vi "AssetMgrChangeHardwareForDeviceRequest_Parse.vi"(8 "error in (no error)":errorcluster, 11 "Message":T17) -> (0 "error out":errorcluster, 1 "Body":T1, 2 "Header":T16, 3 "AssetMgrChangeHardwareForDeviceRequest":T15)   [LabVIEW 2017]
uses:
  <vilib>/addons/InsightCM/MessageBus/Base/controls/Message.ctl
  <vilib>/addons/InsightCM/MessageBus/Base/controls/MessageHeader.ctl
  <vilib>/addons/InsightCM/MessageBus/Base/controls/KeyValuePair.ctl
  <vilib>/addons/InsightCM/MessageBus/MessageLibrary/AssetManager/controls/AssetMgrChangeHardwareForDeviceRequest.ctl
  <vilib>/addons/InsightCM/MessageBus/MessageLibrary/AssetManager/controls/AssetMgrChangeHardwareForDeviceRequestBody.ctl
  <vilib>/addons/InsightCM/MessageBus/Base/controls/DeviceModel.ctl
  <vilib>/addons/InsightCM/MessageBus/Base/controls/Device.ctl
  <vilib>/addons/InsightCM/MessageBus/Base/controls/DeviceState.ctl
  <vilib>/addons/InsightCM/MessageBus/Base/controls/DataGroup.ctl
  <vilib>/addons/InsightCM/MessageBus/Base/controls/BurstModeTrigger.ctl
  <vilib>/addons/InsightCM/MessageBus/Base/controls/Trigger.ctl
  <vilib>/addons/InsightCM/MessageBus/Base/controls/Condition.ctl
  <vilib>/addons/InsightCM/MessageBus/Base/controls/DeviceSensorGroup.ctl
  <vilib>/addons/InsightCM/MessageBus/Base/controls/WirelessEndpoint.ctl
  <vilib>/addons/InsightCM/MessageBus/Base/controls/WirelessChannel.ctl
  <vilib>/addons/InsightCM/MessageBus/Base/controls/Channel.ctl
  <vilib>/addons/InsightCM/MessageBus/Base/controls/Tag.ctl
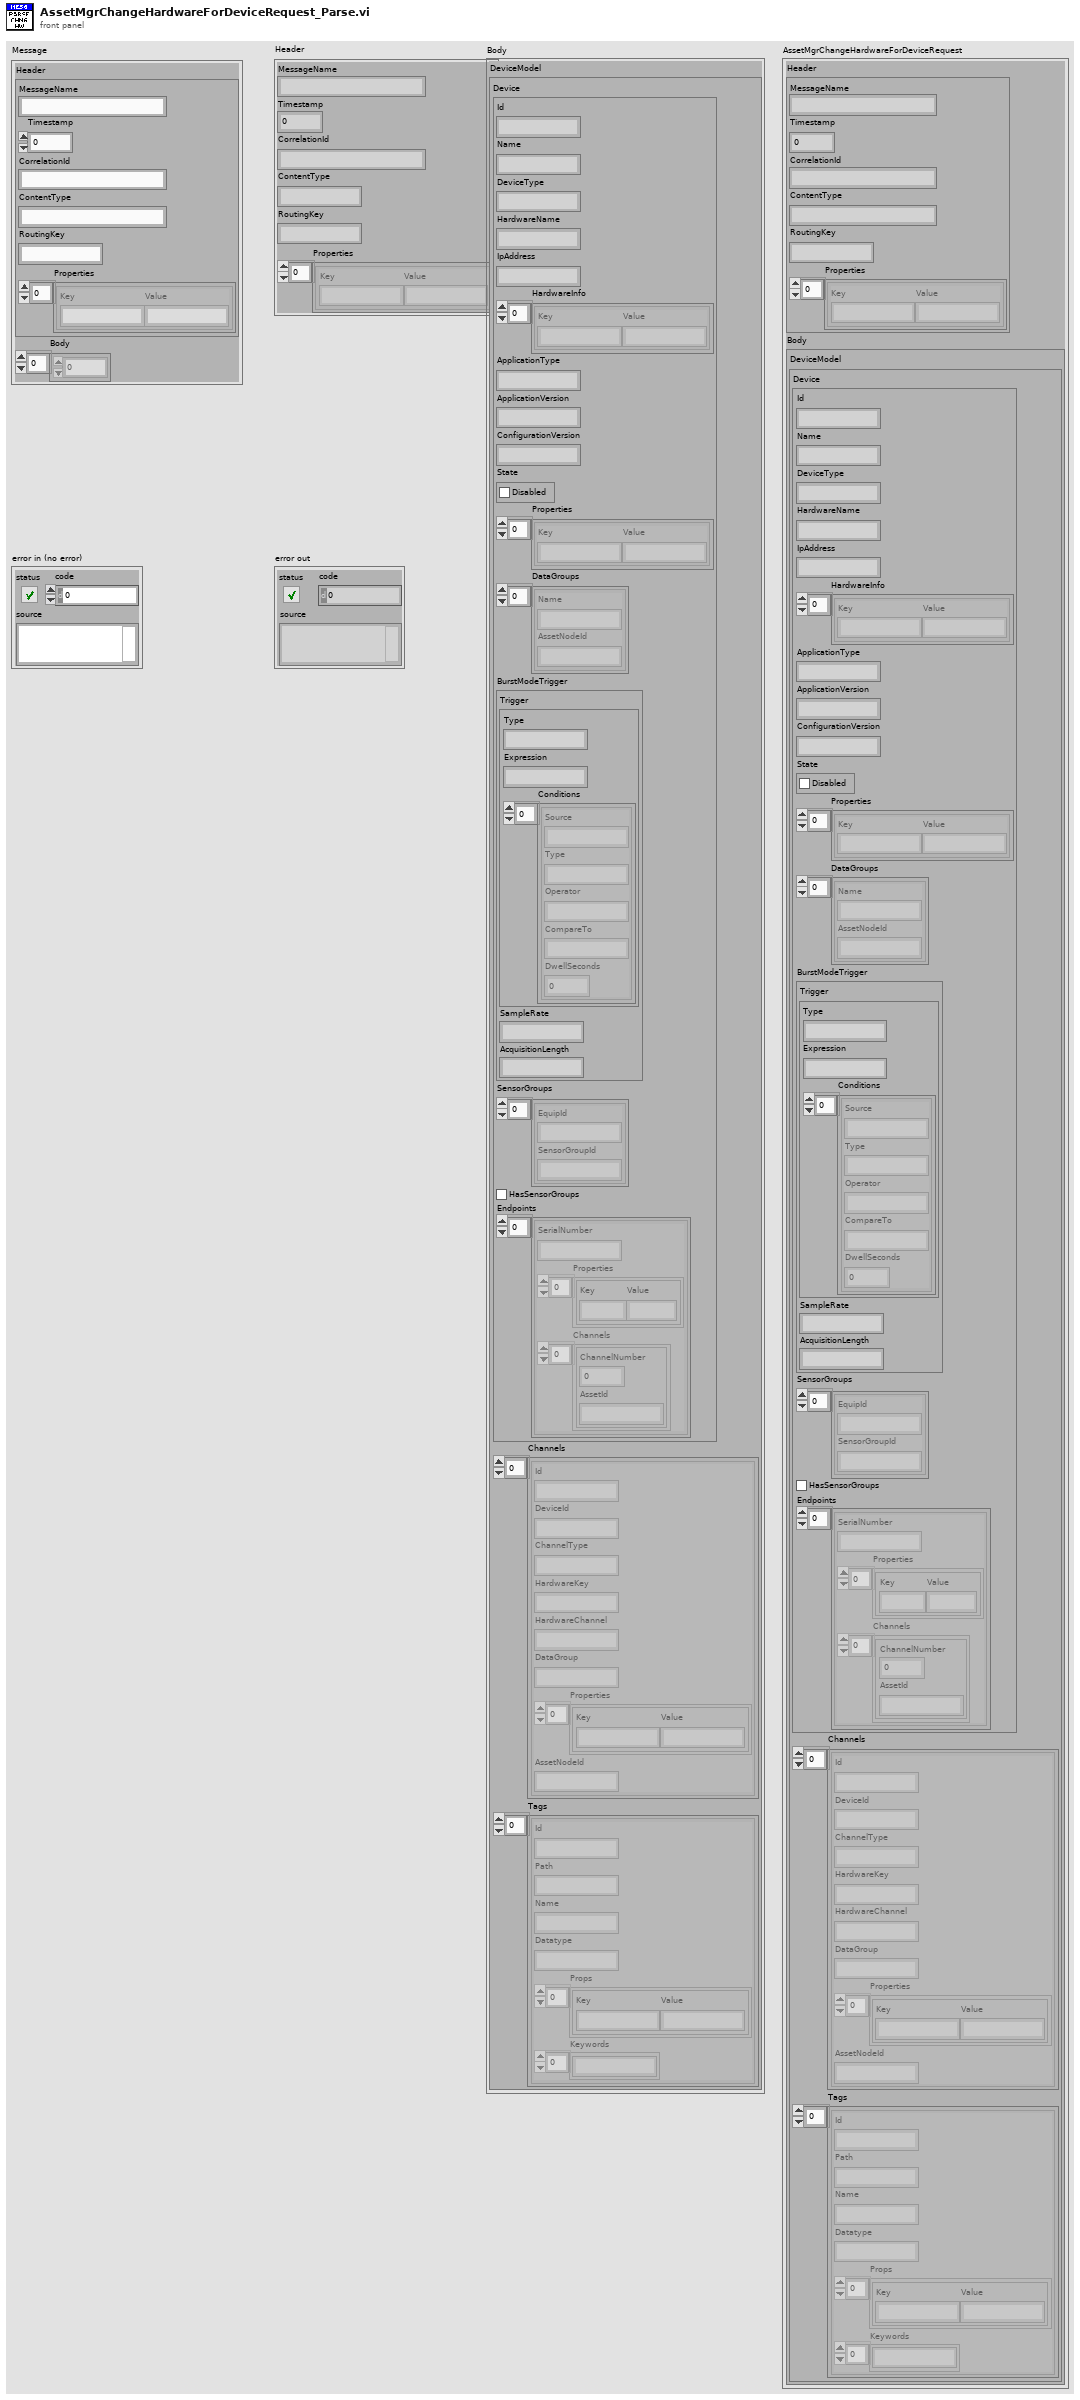
[diagram p1: front panel]
types:
  T1 = typedef "AssetMgrChangeHardwareForDeviceRequestBody.ctl" = cluster{"DeviceModel":T2}
  T2 = typedef "DeviceModel.ctl" = cluster{"Device":T3, "Channels":T13[], "Tags":T14[]}
  T3 = typedef "Device.ctl" = cluster{"Id":string, "Name":string, "DeviceType":string, "HardwareName":string, "IpAddress":string, "HardwareInfo":T4[], "ApplicationType":string, "ApplicationVersion":string, "ConfigurationVersion":string, "State":T5, "Properties":T4[], "DataGroups":T6[], "BurstModeTrigger":T7, "SensorGroups":T10[], "HasSensorGroups":bool, "Endpoints":T11[]}
  T4 = typedef "KeyValuePair.ctl" = cluster{"Key":string, "Value":string}
  T5 = typedef "DeviceState.ctl" = cluster{"Disabled":bool}
  T6 = typedef "DataGroup.ctl" = cluster{"Name":string, "AssetNodeId":string}
  T7 = typedef "BurstModeTrigger.ctl" = cluster{"Trigger":T8, "SampleRate":string, "AcquisitionLength":string}
  T8 = typedef "Trigger.ctl" = cluster{"Type":string, "Expression":string, "Conditions":T9[]}
  T9 = typedef "Condition.ctl" = cluster{"Source":string, "Type":string, "Operator":string, "CompareTo":string, "DwellSeconds":dbl}
  T10 = typedef "DeviceSensorGroup.ctl" = cluster{"EquipId":string, "SensorGroupId":string}
  T11 = typedef "WirelessEndpoint.ctl" = cluster{"SerialNumber":string, "Properties":T4[], "Channels":T12[]}
  T12 = typedef "WirelessChannel.ctl" = cluster{"ChannelNumber":i32, "AssetId":string}
  T13 = typedef "Channel.ctl" = cluster{"Id":string, "DeviceId":string, "ChannelType":string, "HardwareKey":string, "HardwareChannel":string, "DataGroup":string, "Properties":T4[], "AssetNodeId":string}
  T14 = typedef "Tag.ctl" = cluster{"Id":string, "Path":string, "Name":string, "Datatype":string, "Props":T4[], "Keywords":string[]}
  T15 = typedef "AssetMgrChangeHardwareForDeviceRequest.ctl" = cluster{"Header":T16, "Body":T1}
  T16 = typedef "MessageHeader.ctl" = cluster{"MessageName":string, "Timestamp":i64, "CorrelationId":string, "ContentType":string, "RoutingKey":string, "Properties":T4[]}
  T17 = typedef "Message.ctl" = cluster{"Header":T16, "Body":u8[]}
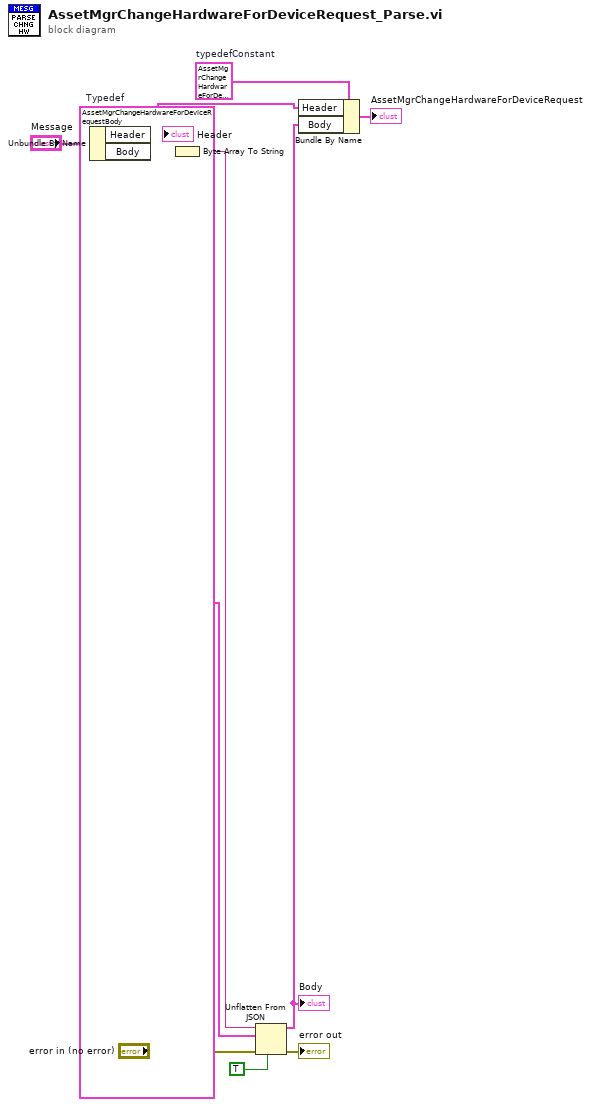
[diagram p0: block diagram]
diagram:
  w3 = T15 {"Header"={"MessageName"="", "Timestamp"=0, "CorrelationId"="", "ContentType"="", "RoutingKey"="", "Properties"=[]}, "Body"={"DeviceModel"={"Device"={"Id"="", "Name"="", "DeviceType"="", "HardwareName"="", "IpAddress"="", "HardwareInfo"=[], "ApplicationType"="", "ApplicationVersion"="", "ConfigurationVersion"="", "State"={"Disabled"=FALSE}, "Properties"=[], "DataGroups"=[], "BurstModeTrigger"={"Trigger"={"Type"="", "Expression"="", "Conditions"=[]}, "SampleRate"="", "AcquisitionLength"=""}, "SensorGroups"=[], "HasSensorGroups"=FALSE, "Endpoints"=[]}, "Channels"=[], "Tags"=[]}}}  # typedefConstant
  w7 = T1 {"DeviceModel"={"Device"={"Id"="", "Name"="", "DeviceType"="", "HardwareName"="", "IpAddress"="", "HardwareInfo"=[], "ApplicationType"="", "ApplicationVersion"="", "ConfigurationVersion"="", "State"={"Disabled"=FALSE}, "Properties"=[], "DataGroups"=[], "BurstModeTrigger"={"Trigger"={"Type"="", "Expression"="", "Conditions"=[]}, "SampleRate"="", "AcquisitionLength"=""}, "SensorGroups"=[], "HasSensorGroups"=FALSE, "Endpoints"=[]}, "Channels"=[], "Tags"=[]}}  # Typedef
  n1 = Unbundle By Name("Message") -> ("Header"=w9:T16, "Body"=w1:u8[])
  "Header" <- w9
  n2 = Byte Array To String(unsigned byte array=w1) -> (string=w6:string)
  n3 = Unflatten From JSON(JSON string=w6, type and defaults=w7, default null elements? (F)=TRUE, error in (no error)="error in (no error)") -> (value=w5:T1, error out=→"error out":errorcluster)  [unwired: 3 in]
  "Body" <- w5
  n4 = Bundle By Name(cluster=w3, "Header"=w9, "Body"=w5) -> (→"AssetMgrChangeHardwareForDeviceRequest":T15)
